vi "PixelValue.vi"(9 "point(x,y)":cluster{"x":i16, "y":i16}, 11 "Picture":picture) -> (3 "Color":u32)   [LabVIEW 2021]
uses:
  vi.lib/LabVIEW Icon API/lv_icon/lv_icon.lvlib
panel:
  out "Color Box":u32(colorbox)
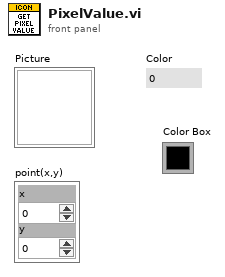
[diagram p1: front panel]
types:
  T1 = cluster{"left":i16, "top":i16, "right":i16, "bottom":i16}
  T2 = typedef "imagedata.ctl" = cluster{"image type":i32, "image depth":i32, "image":u8[], "mask":u8[], "colors":u32[], "Rectangle":cluster{"left":i16, "top":i16, "right":i16, "bottom":i16}}
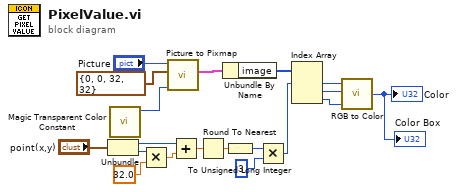
[diagram p0: block diagram]
diagram:
  n1 = Unbundle("point(x,y)") -> ("x"=w11:i16, "y"=w4:i16)
  n2 = call "Magic Transparent Color Constant.vi"() -> ("Magic transparent color constant"=w2:u32)  [unwired: 11 out]
  n3 = Multiply(x=w4, y=32.0) -> (x*y=w3:dbl)
  n4 = call <vilib>:"Picture to Pixmap.vi"("Background Color"=w2, "rect"=T1 {"left"=0, "top"=0, "right"=32, "bottom"=32}, "picture"="Picture") -> ("image data"=w12:T2)  [unwired: 1 in, 7 out]
  n5 = Add(x=w11, y=w3) -> (x+y=w8:dbl)
  n6 = Round To Nearest(number=w8) -> (nearest integer value=w7:dbl)
  n7 = Unbundle By Name(w12) -> ("image"=w13:u8[])
  n8 = To Unsigned Long Integer(number=w7) -> (unsigned 32bit integer=w10:u32)
  n9 = Multiply(x=w10, y=u32 3) -> (x*y=w14:u32)
  n10 = Index Array(array=w13, index #1=w14) -> (element #1=w15:u8, element #2=w16:u8, element #3=w17:u8)  [unwired: 2 in]
  n11 = call <vilib>:"RGB to Color.vi"("B"=w17, "G"=w16, "R"=w15) -> ("Color"=→"Color" →"Color Box":u32)
